vi "Get Events.vi"(11 "Duplicated Channel Dialog View in":refnum<class "Duplicated Channel Dialog View.lvclass">) -> (2 "Events":T1, 3 "Duplicated Channel Dialog View out":refnum<class "Duplicated Channel Dialog View.lvclass">)   [LabVIEW 2013, in "Duplicated Channel Dialog View.lvlib" / "Duplicated Channel Dialog View.lvclass"]
uses:
  Duplicated Channel Dialog View.lvclass
  Typedef/Events.ctl
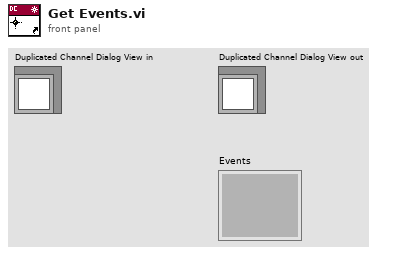
[diagram p1: front panel]
types:
  T1 = typedef "Duplicated Channel Dialog View.lvlib/Duplicated Channel Dialog View.lvclass/Events.ctl" = cluster{}
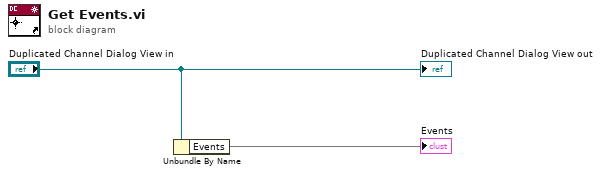
[diagram p0: block diagram]
diagram:
  n1 = Unbundle By Name("Duplicated Channel Dialog View in") -> ("Events"=→"Events")
  "Duplicated Channel Dialog View out" <- "Duplicated Channel Dialog View in"
